vi "CLSUIP_CopyExecutionProperties.vi"(8 "error in (no error)":errorcluster, 10 "Old VI in":refnum<vi>, 11 "New VI in":refnum<vi>) -> (0 "error out":errorcluster, 3 "New VI out":refnum<vi>)   [LabVIEW 2021, in "MemberVICreation.lvlib" / "VIRetooler.lvclass"]
uses:
  <resource>/Framework/Providers/LVClassLibrary/NewAccessors/VIRetooler/VIRetooler.lvclass
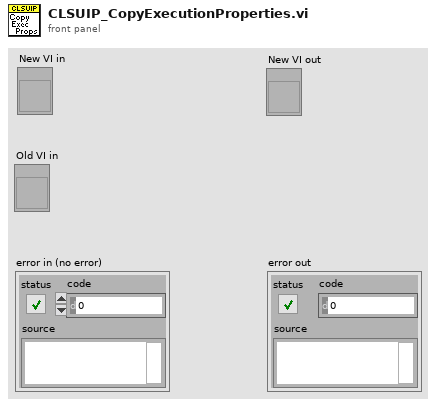
[diagram p1: front panel]
types:
  T1 = enum32{"invalid execution system", "user interface", "standard", "instrument i/o", "data acquisition", "other 1", "other 2", "same as caller"}
  T2 = enum32{"invalid priority", "background priority", "normal priority", "above normal priority", "high priority", "time critical priority", "subroutine"}
  T3 = enum16{"Share clones between instances", "Preallocate clone for each instance"}
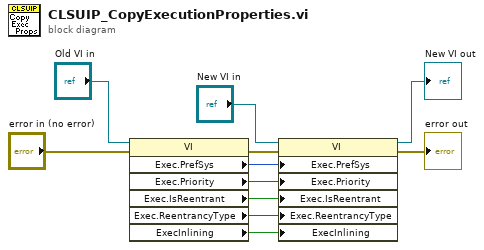
[diagram p0: block diagram]
diagram:
  n1 = property class="VI"(reference="Old VI in", error in="error in (no error)") -> (error out=w4:errorcluster, "Exec.PrefSys"=w11:T1, "Exec.Priority"=w10:T2, "Exec.IsReentrant"=w9:bool, "Exec.ReentrancyType"=w5:T3, "ExecInlining"=w1:bool)  [unwired: 1 out]
  n2 = property class="VI"(reference="New VI in", error in=w4, "Exec.PrefSys"=w11, "Exec.Priority"=w10, "Exec.IsReentrant"=w9, "Exec.ReentrancyType"=w5, "ExecInlining"=w1) -> (reference out=→"New VI out":refnum<vi>, error out=→"error out":errorcluster)
